vi "Signal Number Control.vi"(9 "init":bool, 10 "Previous PMT1":bool, 11 "PMT1_signal in":u16) -> (1 "output":bool, 2 "IO Module\\PMT1":bool, 3 "PMT1_signal out":u16)   [LabVIEW 2015]
uses:
  <vilib>/rvi/eio/common/nirviEmuTemplateMethod_errors.vi
  Grobal Variable_Pixel Clock.vi
  <vilib>/eio/EIONode/EIONode.xnode
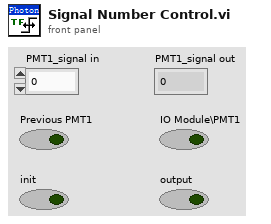
[diagram p1: front panel]
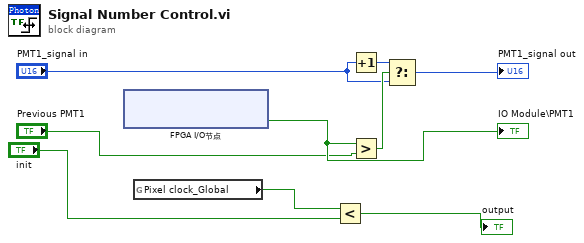
[diagram p0: block diagram]
diagram:
  n1 = xnode "FPGA I/O节点"() -> ("IO Module\\PMT1"=w9:bool)  [unwired: 1 in, 1 out]
  "IO Module\\PMT1" <- w9
  n2 = global read "Grobal Variable_Pixel Clock.vi" "Pixel clock_Global"() -> (w5:bool)
  n3 = Less?(x=w5, y="init") -> (x < y?=→"output":bool)
  n4 = Increment(x="PMT1_signal in") -> (x+1=w2:u16)
  n5 = Greater?(x=w9, y="Previous PMT1") -> (0:w8:bool)
  n6 = Select(t=w2, s=w8, f="PMT1_signal in") -> (s? t:f=→"PMT1_signal out":u16)
